vi "Parce Response.vi"(8 "error in":errorcluster, 11 "MES Response":string="<?xml version=\"1.0\" encoding=\"utf-8\"?>\n<soap:Envelope xmlns:xsi=\"http://www.w3.org/2001/XMLSchema-instance\" xmlns:xsd=\"http://www.w3.org/2001/XMLSchema\" xmlns:soap=\"http://schemas.xmlsoap.org/soap/envelope/\">\n  <soap:Body>\n    <ExecuteResponse xmlns=\"http://tempuri.org/\">\n      <ExecuteResult>\n        <Result>string</Result>\n        <MessageCode>string</MessageCode>\n        <MessageDescription>string</MessageDescription>\n        <BoxNo>string</BoxNo>\n        <PalletNo>string</PalletNo>\n        <PackingInstruction1>string1</PackingInstruction1>\n        <PackingInstruction2>string2</PackingInstruction2>\n        <PackingInstruction3>string3</PackingInstruction3>\n        <PackingInstruction4>string4</PackingInstruction4>\n        <PackingInstruction5>string</PackingInstruction5>\n        <SerialCount>int</SerialCount>\n        <MaxSerialCount>int</MaxSerialCount>\n        <BoxCount>int</BoxCount>\n        <MaxBoxCount>int</MaxBoxCount>\n      </ExecuteResult>\n    </ExecuteResponse>\n  </soap:Body>\n</soap:Envelope>\n") -> (0 "error out":errorcluster)   [LabVIEW 2023, in "MES.lvlib"]
uses:
  MES.lvlib
panel:
  out "concatenated string":string
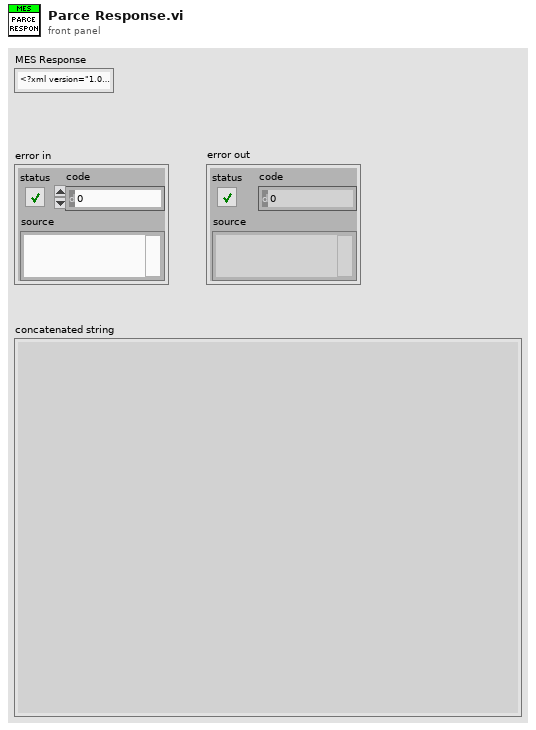
[diagram p1: front panel]
types:
  T1 = enum16{"open", "replace", "create", "open or create", "replace or create", "replace or create with confirmation"}
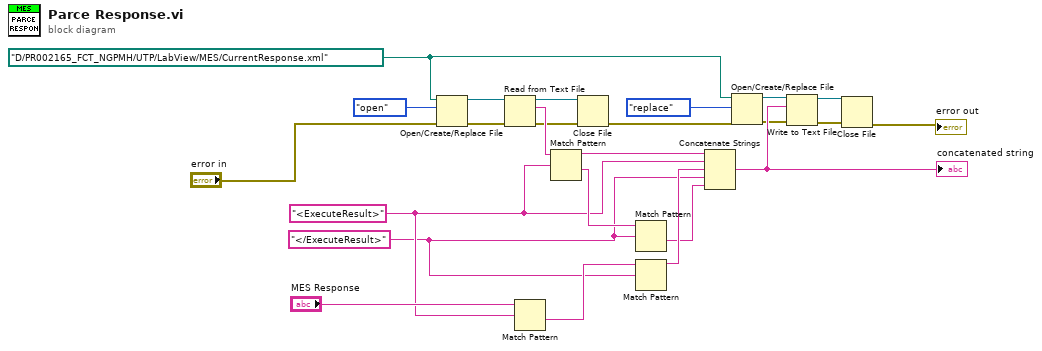
[diagram p0: block diagram]
diagram:
  w13 = "</ExecuteResult>" ("regular expression")
  w15 = "<ExecuteResult>" ("regular expression")
  w7 = path "D:/PR002165_FCT_NGPMH/UTP/LabView/MES/CurrentResponse.xml" ("file path (use dialog)")
  n1 = Open/Create/Replace File(file path (use dialog)=w7, error in="error in", operation (0:open)=T1."open") -> (refnum out=w24:refnum<file>, error out=w11:errorcluster)  [unwired: 3 in, 1 out]
  n2 = Read from Text File(file (use dialog)=w24, error in=w11) -> (refnum out=w17:refnum<file>, text=w23:string, error out=w10:errorcluster)  [unwired: 2 in, 1 out]
  n3 = Match Pattern(string="MES Response", regular expression=w15) -> (after substring=w21:string)  [unwired: 1 in, 3 out]
  n4 = Match Pattern(string=w23, regular expression=w15) -> (before substring=w14:string, after substring=w19:string)  [unwired: 1 in, 2 out]
  n5 = Close File(refnum=w17, error in=w10) -> (error out=w3:errorcluster)  [unwired: 1 out]
  n6 = Match Pattern(string=w19, regular expression=w13) -> (after substring=w12:string)  [unwired: 1 in, 3 out]
  n7 = Match Pattern(string=w21, regular expression=w13) -> (before substring=w20:string)  [unwired: 1 in, 3 out]
  n8 = Concatenate Strings(w14, w15, w20, w13, w12) -> (w16:string)
  "concatenated string" <- w16
  n9 = Open/Create/Replace File(file path (use dialog)=w7, error in=w3, operation (0:open)=T1."replace") -> (refnum out=w5:refnum<file>, error out=w2:errorcluster)  [unwired: 3 in, 1 out]
  n10 = Write to Text File(file (use dialog)=w5, text=w16, error in=w2) -> (refnum out=w4:refnum<file>, error out=w1:errorcluster)  [unwired: 1 in, 1 out]
  n11 = Close File(refnum=w4, error in=w1) -> (error out=→"error out":errorcluster)  [unwired: 1 out]
